vi "Get Models.vi"(0 "reference in":refnum<class "Battery.lvclass">, 5 "Error In":errorcluster) -> (14 "reference out":refnum<class "Battery.lvclass">, 16 "models":string[](array[string]), 19 "Error Out":errorcluster)   [LabVIEW 2023, in "Battery.lvclass"]
uses:
  Battery.lvclass
  Battery.lvclass/Battery.ctl
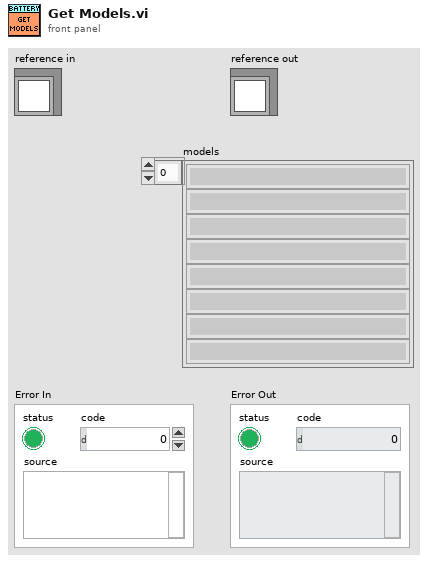
[diagram p1: front panel]
types:
  T1 = typedef "Battery.lvclass/ObjectAttributes.ctl" = cluster{"Python module":path, "Python Session":refnum<k35>, "PybammWrapper":refnum<k38>, "model loaded":bool, "simulation loaded":bool, "OCV SOC Curve":dbl[][]}
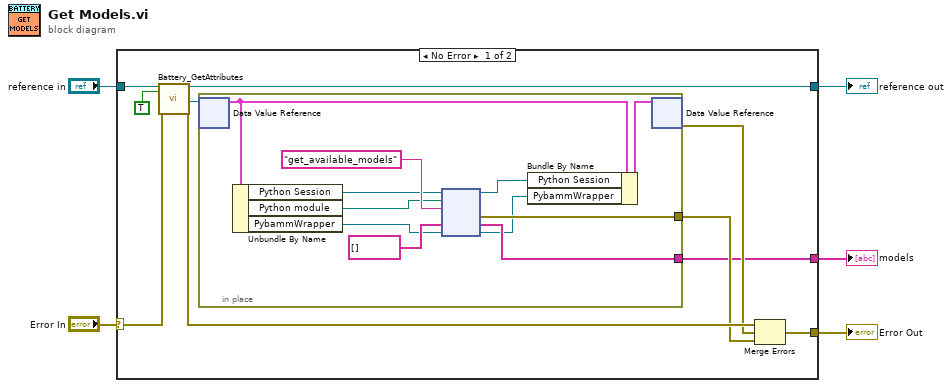
[diagram p0: block diagram]
diagram:
  n1 = case shown="No Error" "Error In" {
    selector: "Error In" -> [w14 w28]
    tunnel: [w12 w28] -> w4
    tunnel: [w13 w27] -> w2
    tunnel: "reference in" -> [w15 w27]
    tunnel: [w6 _] -> w1
    frame No Error {
      n2 = call "Battery_GetAttributes.vi"("reference in"=w15, "OnlyGetDvrReference(False)"=TRUE, "Error In"=w14) -> ("reference out"=w13:refnum<class "Battery.lvclass">, "DataRef"=w11:refnum<data-value>, "Error Out"=w9:errorcluster)  [unwired: 13 in, 1 out]
      n3 = in-place {
        in-place-border: [w21] -> w7
        in-place-border: [w20] -> w6
        n4 = in-place-dvr #1(w11) -> (w19:T1)  [unwired: 1 out]
        n5 = Unbundle By Name(w19) -> ("Python Session"=w23:refnum<k35>, "Python module"=w22:path, "PybammWrapper"=w24:refnum<k38>)
        n6 = node(w23, w22, "get_available_models" ("function name"), string[] [], w24) -> (w16:refnum<k35>, w21:errorcluster, w20:string[], w17:refnum<k38>)  [unwired: 1 in, 2 out]
        n7 = Bundle By Name(cluster=w19, "Python Session"=w16, "PybammWrapper"=w17) -> (w18:T1)
        n8 = in-place-dvr #1(w18) -> (w8:errorcluster)  [unwired: 1 out]
      }
      n9 = Merge Errors(w9, w8, w7) -> (w12:errorcluster)
    }
    frame Error {
    }
  }
  "Error Out" <- w4
  "reference out" <- w2
  "models" <- w1
